vi "_ConvertVialNumber.vi"(0 "Vial#":string) -> (2 "NumericVial#":u16, 3 "NumericVial# 2":string, 4 "Valid":bool)   [LabVIEW 2012]
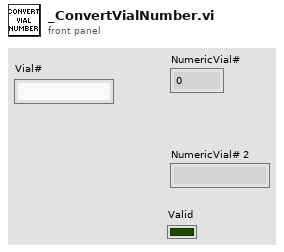
[diagram p1: front panel]
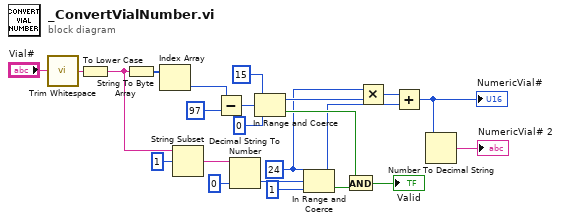
[diagram p0: block diagram]
diagram:
  w6 = u16 24 ("upper limit")
  n1 = call <vilib>:"Trim Whitespace.vi"("string"="Vial#") -> ("trimmed string"=w22:string)  [unwired: 1 in]
  n2 = To Lower Case(string=w22) -> (all lower case string=w19:string)
  n3 = String To Byte Array(string=w19) -> (unsigned byte array=w23:u8[])
  n4 = Index Array(array=w23) -> (element=w18:u8)  [unwired: 1 in]
  n5 = String Subset(string=w19, offset (0)=1) -> (substring=w13:string)  [unwired: 1 in]
  n6 = Subtract(x=w18, y=u8 97) -> (x-y=w16:u8)
  n7 = Decimal String To Number(string=w13, default (0L)=u16 0 ("default (0 I32)")) -> (number=w12:u16)  [unwired: 1 in, 1 out]
  n8 = In Range and Coerce(upper limit=u8 15, x=w16, lower limit=u8 0) -> (coerced(x)=w7:u8, In Range?=w9:bool)
  n9 = In Range and Coerce(upper limit=w6, x=w12, lower limit=u16 1) -> (coerced(x)=w4:u16, In Range?=w10:bool)
  n10 = And(x=w9, y=w10) -> (x .and. y?=→"Valid":bool)
  n11 = Multiply(x=w6, y=w7) -> (x*y=w5:u16)
  n12 = Add(x=w5, y=w4) -> (x+y=w1:u16)
  "NumericVial#" <- w1
  n13 = Number To Decimal String(number=w1) -> (decimal integer string=→"NumericVial# 2":string)  [unwired: 1 in]
